vi "1905x Series Delay.vi"(8 "error in (no error)":errorcluster, 9 "milliseconds to wait":dbl min=0.0 max=1000.0 format="%.3f") -> (0 "error out":errorcluster)   [LabVIEW 2015]
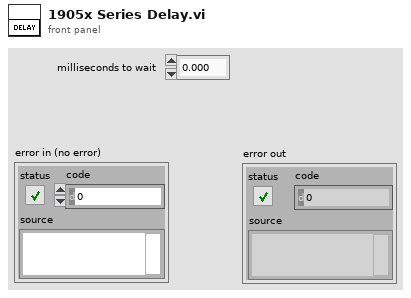
[diagram p1: front panel]
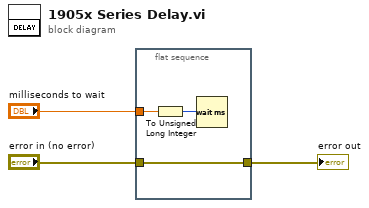
[diagram p0: block diagram]
diagram:
  n1 = flat-sequence {
    tunnel: "milliseconds to wait" -> [w6]
    tunnel: "error in (no error)" -> [w4]
    tunnel: [w4] -> w1
    frame #0 {
      n2 = To Unsigned Long Integer(number=w6) -> (unsigned 32bit integer=w5:u32)
      n3 = Wait (ms)(milliseconds to wait=w5) -> ()  [unwired: 1 out]
    }
  }
  "error out" <- w1
